vi "Cannont Claim Address.vi"(0 "session out":refnum<k21>, 7 "Names":T1[](array[typedef]), 11 "error in":errorcluster) -> (15 "error out":errorcluster)   [LabVIEW 2015, in "J1939 Addon Engine.lvlib"]
uses:
  J1939 Addon Engine.lvlib
  Shared/J1939 Utilities/Types/Convert CAN Data (U8) Cluster.ctl
  Shared/J1939 Utilities/Types/CAN Outgoing Message Cluster.ctl
  Shared/J1939 Utilities/Types/PGN Fields Cluster.ctl
  Shared/J1939 Utilities/SubVIs/Convert J1939 ID to CAN Arb ID.vi
  <vilib>/xnet/xnet.llb/XNET Write (Frame CAN).vi
  Shared/J1939 Utilities/J1939 Utilities.lvlib
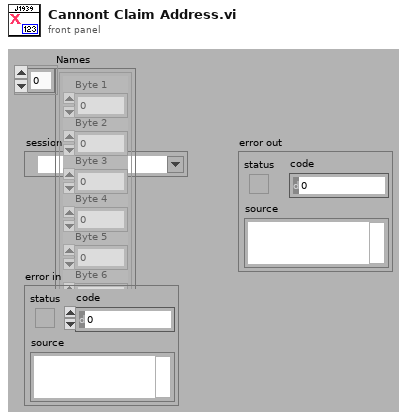
[diagram p1: front panel]
types:
  T1 = typedef "J1939 Addon Shared.lvlib/J1939 Utilities.lvlib/Convert CAN Data (U8) Cluster.ctl" = cluster{"Byte 1":u8, "Byte 2":u8, "Byte 3":u8, "Byte 4":u8, "Byte 5":u8, "Byte 6":u8, "Byte 7":u8, "Byte 8":u8}
  T2 = typedef "J1939 Addon Shared.lvlib/J1939 Utilities.lvlib/PGN Fields Cluster.ctl" = cluster{"Reserved Bit":u8, "Data page":u8, "PDU Format":u8, "PDU Specific":u8}
  T3 = typedef "J1939 Addon Shared.lvlib/J1939 Utilities.lvlib/CAN Outgoing Message Cluster.ctl" = cluster{"Identifier":u32, "Data":u8[]}
  T4 = typedef "XNET Frame CAN.ctl" = cluster{"timestamp":timestamp, "payload":u8[], "identifier":u32, "type":T5, "extended?":bool, "echo?":bool}
  T5 = typedef "XNET Frame Type CAN.ctl" = u8
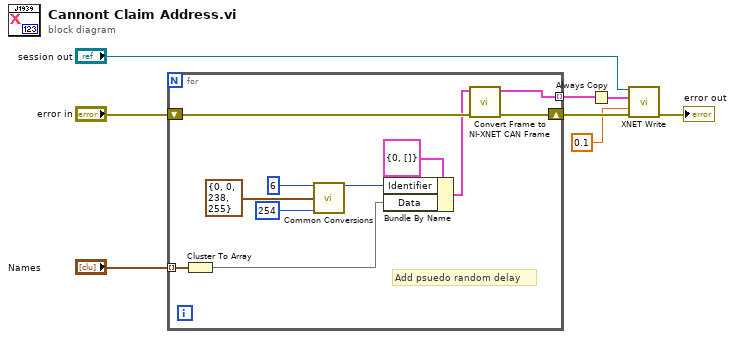
[diagram p0: block diagram]
diagram:
  n1 = for {
    tunnel: "Names" -> [w19] mode=indexing
    tunnel: [w10] -> w3 mode=indexing
    shift-right: [w18] -> w5
    shift-left: "error in" -> [w17]
    # "Add psuedo random delay"
    n2 = Cluster To Array(cluster=w19) -> (array=w9:u8[])
    n3 = call-poly "Common Conversions.vi"("Priority"=u8 6, "PGN Fields"=T2 {"Reserved Bit"=0, "Data page"=0, "PDU Format"=238, "PDU Specific"=255}, "Source Address"=u8 254) -> ("ID"=w12:u32)  [unwired: 2 in, 10 out]
    n4 = Bundle By Name(cluster=T3 {"Identifier"=0, "Data"=[]} ("Data to Send"), "Identifier"=w12, "Data"=w9) -> (w16:T3)
    n5 = call "Convert Frame to NI-XNET CAN Frame.vi"("error in (no error)"=w17, "Data to Send"=w16) -> ("error out"=w18:errorcluster, "CAN frame"=w10:T4)  [unwired: 8 in]
  }
  n6 = Always Copy(1:w3) -> (0:w1:T4[])
  n7 = call-poly <vilib>:"XNET Write.vi"("session in"="session out", "data"=w1, "timeout (10)"=0.1, "error in (no error)"=w5) -> ("error out"=→"error out":errorcluster)  [unwired: 11 out]
